vi "BRig_dataLC_Loop2_T.vi"() -> (2 "output_Loop2_T":i32)   [LabVIEW 2014]
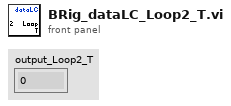
[diagram p1: front panel]
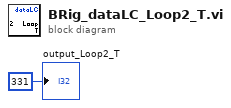
[diagram p0: block diagram]
diagram:
  "output_Loop2_T" <- 331 ("output_iBlock")
